vi "Read Waveform (Single).vi"(8 "error in (no error)":errorcluster, 9 "Timeout (10000 ms)":u32=10000, 10 "Source (1: Channel 1)":u16(ring)=1 items=["Channel 1"=1, "Channel 2"=2, "Channel 3"=3, "Channel 4"=4], 11 "VISA resource name":refnum<visa-resource-name>) -> (0 "error out":errorcluster, 2 "Waveform Data":waveform(dbl)(graph), 3 "VISA resource name out":refnum<visa-resource-name>)   [LabVIEW 2021, in "Siglent SDS 1000 2000 Series.lvlib"]
doc: "Initiates an acquisition on all channels that you enabled with the <B>Configure Channel</B> VI. The VI waits for the acquisition to complete and returns the waveform for the Source channel you specified. If the oscilloscope did not complete the acquisition within the time period you specify with the Timeout parameter, the VI returns a time out error. A common cause for a timeout error is the acquisition was not triggered. For example, the trigger level is out of range of the waveform.\n\nCall the <B>Fetch Waveform</B> VI to obtain the waveforms for each of the remaining enabled Source channels without initiating another acquisition.\n\nNote: If your instrument does not support auto compensation for probe attenuation, you may need to adjust the scaling of the Waveform Data accordingly. This is handled automatically in the <B>Configure Channel</B> VI or can be done manually by multiplying the Waveform Data by the probe attenuation."
uses:
  <instrlib>/Siglent SDS 1000 2000 Series/Siglent SDS 1000 2000 Series.lvlib
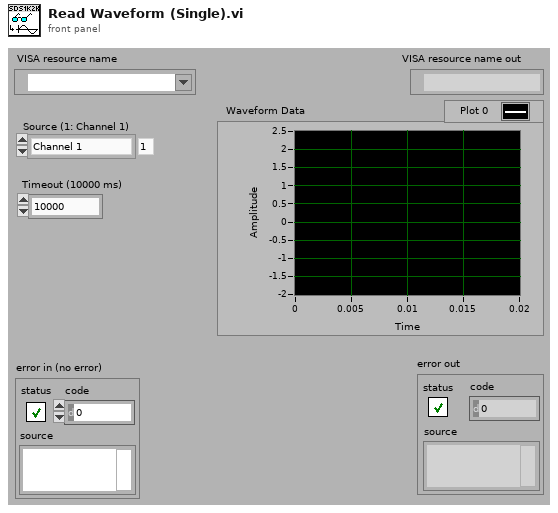
[diagram p1: front panel]
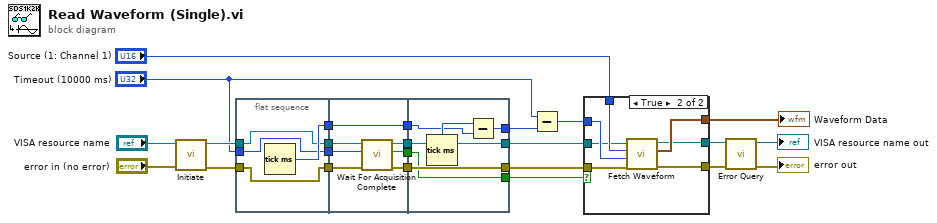
[diagram p0: block diagram]
diagram:
  n1 = call <instrlib>:"Initiate.vi"("error in (no error)"="error in (no error)", "VISA resource name"="VISA resource name") -> ("error out"=w15:errorcluster, "VISA resource name out"=w16:refnum<visa-resource-name>)  [unwired: 8 in]
  n2 = flat-sequence {
    tunnel: "Timeout (10000 ms)" -> [w27]
    tunnel: [w27] -> w8
    tunnel: w16 -> [w26]
    tunnel: [w26] -> w7
    tunnel: w15 -> [w25]
    tunnel: [w25] -> w6
    tunnel: [w28] -> w5
    tunnel: w8 -> [w35]
    tunnel: w7 -> [w33]
    tunnel: w6 -> [w31]
    tunnel: [w30] -> w4
    tunnel: [w32] -> w3
    tunnel: [w34] -> w2
    tunnel: w5 -> [w29]
    tunnel: [w29] -> w1
    tunnel: [w38] -> w14
    tunnel: w4 -> [w38]
    tunnel: [w37] -> w10
    tunnel: w3 -> [w37]
    tunnel: [w39] -> w12
    tunnel: [w36] -> w9
    tunnel: w2 -> [w36]
    tunnel: w1 -> [w40]
    frame #0 {
      n3 = Tick Count (ms)() -> (millisecond timer value=w28:u32)
    }
    frame #1 {
      n4 = call <instrlib>:"Wait For Acquisition Complete.vi"("error in (no error)"=w31, "Timeout (10000 ms)"=w35, "VISA resource name"=w33) -> ("error out"=w30:errorcluster, "Complete"=w34:bool, "VISA resource name out"=w32:refnum<visa-resource-name>)  [unwired: 6 in]
    }
    frame #2 {
      n5 = Tick Count (ms)() -> (millisecond timer value=w41:u32)
      n6 = Subtract(x=w41, y=w40) -> (x-y=w39:u32)
    }
  }
  n7 = Subtract(x="Timeout (10000 ms)", y=w12) -> (x-y=w11:u32)
  n8 = case shown="True" w9 {
    tunnel: [_ w50] -> w22
    tunnel: [w43 w49] -> w21
    tunnel: [w42 w48] -> w19
    tunnel: "Source (1: Channel 1)" -> [_ w47]
    tunnel: w14 -> [w42 w46]
    tunnel: w11 -> [_ w45]
    tunnel: w10 -> [w43 w44]
    frame False {
    }
    frame True {
      n9 = call <instrlib>:"Fetch Waveform.vi"("error in (no error)"=w46, "Timeout (10000 ms)"=w45, "Source (1: Channel 1)"=w47, "VISA resource name"=w44) -> ("error out"=w48:errorcluster, "Waveform Graph"=w50:waveform(dbl), "VISA resource name out"=w49:refnum<visa-resource-name>)  [unwired: 5 in]
    }
  }
  "Waveform Data" <- w22
  n10 = call <instrlib>:"Error Query.vi"("error in (no error)"=w19, "VISA resource name"=w21) -> ("error out"=→"error out":errorcluster, "VISA resource name out"=→"VISA resource name out":refnum<visa-resource-name>)  [unwired: 6 in, 2 out]
